vi "random_array_1D.vi"(8 "offset":dbl format="%#_13g", 9 "scale":dbl=0.1 format="%#_13g", 11 "N":i32=100) -> (2 "Array":dbl[](array[numeric])=[0.04930690809012457, 0.09596777003171647, 0.03865812475340505, 0.05962222269139579, 0.007050006098414264, 0.00612620918636364, 0.000456234047370141, 0.04321813538056751, 0.04012053244751406, 0.08904750397450684, 0.0336504308663095, 0.004586250885604981, 0.05142294306959359, 0.06521838984066648, 0.07150009765212935, 0.06422218331814512, 0.07235272815528586, 0.06684906211950313, 0.05302768763866261, 0.0046620670406394725, 0.08138535341639705, 0.044142182256147855, 0.08065298324753481, 0.05696465403409967, 0.05883910871468112, 0.07343859524517656, 0.03846135124211021, 0.047358844035739936, 0.0022030224100495267, 0.012298593873745656, 0.07017926395940277, 0.04488176252792464, 0.02026361323222017, 0.004228685721116898, 0.012545942359666329, 0.06400523278105107, 0.07728175536675044, 0.09214650968903702, 0.08512975492790242, 0.06354530315411866, 0.08068430520089465, 0.049794991617851996, 0.013792586385366335, 0.01271879568707679, 0.06136821508538104, 0.04732936401026344, 0.024587228923879836, 0.016934238260578407, 0.05959444458448764, 0.09480993351230918, 0.06230047378631101, 0.04985570716784418, 0.013775180662099151, 0.08527400838054065, 0.08923576614328602, 0.025702595919040335, 0.09841712353373451, 0.00501223852210635, 0.03206677400834268, 0.021021043945266008, 0.015346056759296102, 0.017222824628023714, 0.009086082971813948, 0.03817729586191834, 0.04763542743445762, 0.026529063273474596, 0.04084547990689602, 0.013832101886590476, 0.026209778985838962, 0.09932860053484323, 0.04405690646227556, 0.041017251853431816, 0.05771975455682641, 0.08945463722272609, 0.09787689452181492, 0.05273475196187949, 0.06028563311742901, 0.016303044645927446, 0.056353052188848146, 0.05044581254982277, 0.05160915101403057, 0.08299230285216873, 0.09768772617275717, 0.08244892202053784, 0.06753462753281532, 0.09929927142655365, 0.07598937812774137, 0.0909120772051886, 0.026771109808852958, 0.07455657027208158, 0.05473492845851189, 0.047449548826339207, 0.017847529102433545, 0.01814998321981545, 0.032107117180310674, 0.07753643661122554, 0.01775709634456999, 0.028284255375911328, 0.006331061552791284, 0.08839119456881442])   [LabVIEW 2015, in "daq_simulate.lvlib"]
uses:
  daq_simulate.lvlib
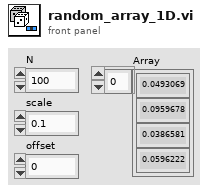
[diagram p1: front panel]
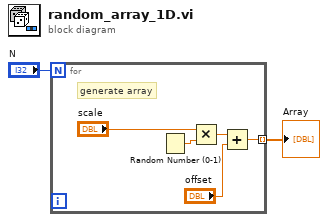
[diagram p0: block diagram]
diagram:
  n1 = for {
    N: "N" -> [_]
    tunnel: [w7] -> w1 mode=indexing
    # "generate array"
    n2 = Random Number (0-1)() -> (number: 0 to 1=w6:dbl)
    n3 = Multiply(x="scale", y=w6) -> (x*y=w4:dbl)
    n4 = Add(x=w4, y="offset") -> (x+y=w7:dbl)
  }
  "Array" <- w1
